vi "BRig_RT_comm_tcp_write_RTwrite__RunState_Trial_start.vi"(11 "input_dataCurrent":u16[](array[numeric])) -> (2 "output_strCmd":string)   [LabVIEW 2014]
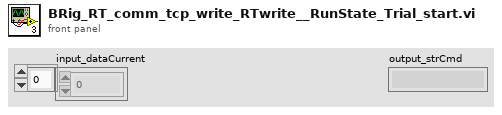
[diagram p1: front panel]
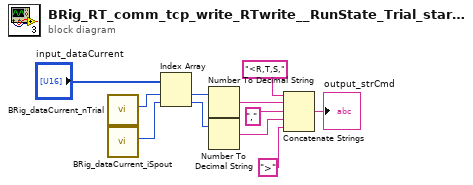
[diagram p0: block diagram]
diagram:
  n1 = call "BRig_dataCurrent_nTrial.vi"() -> ("output_nTrial"=w11:i32)  [unwired: 11 in]
  n2 = call "BRig_dataCurrent_iSpout.vi"() -> ("output_iSpout"=w6:i32)  [unwired: 11 in]
  n3 = Index Array(array="input_dataCurrent", index #1=w11, index #2=w6) -> (element #1=w10:u16, element #2=w5:u16)
  n4 = Number To Decimal String(number=w10) -> (decimal integer string=w9:string)  [unwired: 1 in]
  n5 = Number To Decimal String(number=w5) -> (decimal integer string=w4:string)  [unwired: 1 in]
  n6 = Concatenate Strings("<R,T,S," ("string"), w9, "," ("string"), w4, ">" ("string")) -> (→"output_strCmd":string)
